vi "Align Bottom Row.vi"(8 "error in":errorcluster, 11 "sorted array":cluster{"Rectangle":T1, refnum<vi>}[](array[cluster])) -> (0 "error out":errorcluster)   [LabVIEW 2014]
uses:
  <vilib>/Utility/miscctls.llb/LVRectTypeDef.ctl
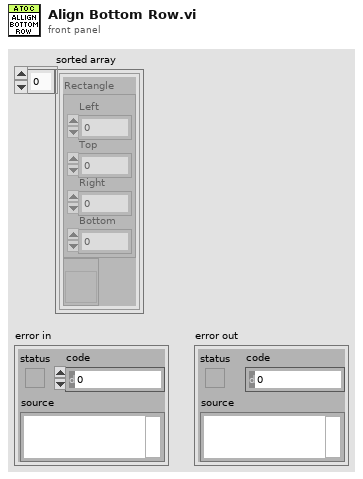
[diagram p1: front panel]
types:
  T1 = typedef "LVRectTypeDef.ctl" = cluster{"Left":i16, "Top":i16, "Right":i16, "Bottom":i16}
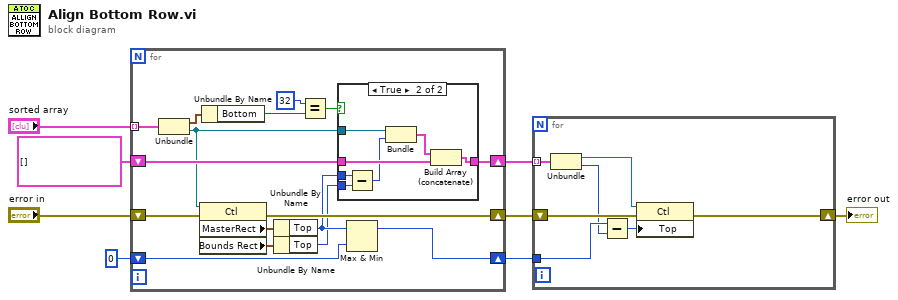
[diagram p0: block diagram]
diagram:
  n1 = for {
    shift-right: [w18] -> w3
    shift-left: cluster{refnum<vi>, i16}[] [] -> [w22]
    tunnel: "sorted array" -> [w20] mode=indexing
    shift-right: [w12] -> w4
    shift-left: 0 -> [w15]
    shift-right: [w13] -> w2
    shift-left: "error in" -> [w14]
    n2 = Unbundle(w20) -> ("Rectangle"=w19:T1, w17:refnum<vi>)
    n3 = property class="Ctl"(reference=w17, error in=w14) -> (error out=w13:errorcluster, "MasterRect"=w16:T1, "Bounds Rect"=w11:T1)  [unwired: 1 out]
    n4 = Unbundle By Name(w19) -> ("Bottom"=w24:i16)
    n5 = Unbundle By Name(w16) -> ("Top"=w10:i16)
    n6 = Unbundle By Name(w11) -> ("Top"=w9:i16)
    n7 = Equal?(x=i16 32 ("y"), y=w24) -> (x = y?=w21:bool)
    n8 = case shown="True" w21 {
      tunnel: [w25 w32] -> w18
      tunnel: w22 -> [w25 w31]
      tunnel: w17 -> [_ w30]
      tunnel: w10 -> [_ w29]
      tunnel: w9 -> [_ w28]
      frame False {
      }
      frame True {
        n9 = Subtract(x=w29, y=w28) -> (x-y=w26:i16)
        n10 = Bundle(w30, w26) -> (w27:cluster{refnum<vi>, i16})  [unwired: 1 in]
        n11 = Build Array (concatenate)(w27, w31) -> (w32:cluster{refnum<vi>, i16}[])
      }
    }
    n12 = Max & Min(x=w10, y=w15) -> (max(x,y)=w12:i32)  [unwired: 1 out]
  }
  n13 = for {
    tunnel: w4 -> [w39]
    tunnel: w3 -> [w38] mode=indexing
    shift-right: [w36] -> w7
    shift-left: w2 -> [w37]
    n14 = Unbundle(w38) -> (w34:refnum<vi>, w33:i16)
    n15 = Subtract(x=w39, y=w33) -> (x-y=w35:i32)
    n16 = property class="Ctl"(reference=w34, error in=w37, "Top"=w35) -> (error out=w36:errorcluster)  [unwired: 1 out]
  }
  "error out" <- w7
